vi "SaveUTCraftFile.vi"(8 "错误输入（无错误）":errorcluster) -> (0 "错误输出":errorcluster)   [LabVIEW 2014]
uses:
  X86Dll/ZXUTConfigMgr.dll
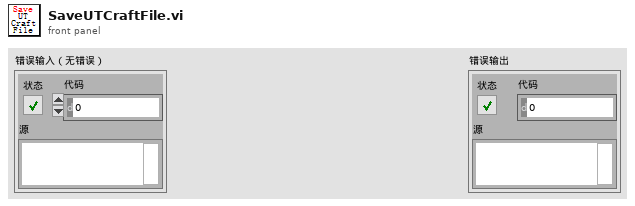
[diagram p1: front panel]
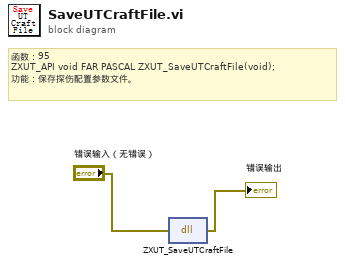
[diagram p0: block diagram]
diagram:
  # "函数：95\nZXUT_API void\tFAR PASCAL ZXUT_SaveUTCraftFile(void);\n功能：保存探伤配置参数文件。"
  n1 = dll-call lib="D:/Software/Utrasonic on-line monitoring/X86Dll/ZXUTConfigMgr.dll" fn="ZXUT_SaveUTCraftFile"(error in="错误输入（无错误）") -> (error out=→"错误输出":errorcluster)  [unwired: 3 in, 1 out]
